vi "Create board.vi"(8 "error in (no error)":errorcluster) -> (0 "error out":errorcluster, 3 "Empty board":refnum<class "Board.lvclass">)   [LabVIEW 2016, in "Chesslib.lvlib" / "Board.lvclass"]
uses:
  Board.lvclass
  Pieces/Piece/Piece.lvclass
  private/Square content.ctl
  Board.lvclass/Board.ctl
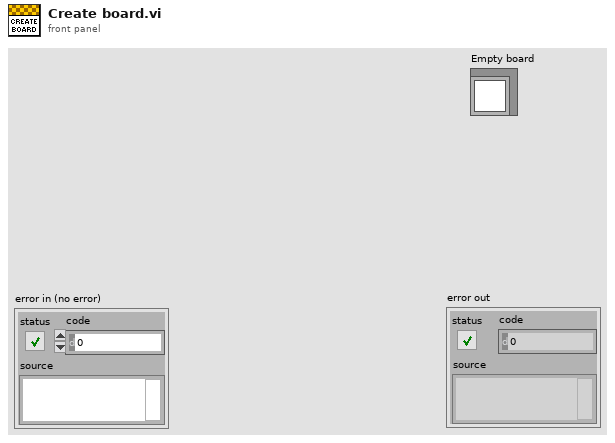
[diagram p1: front panel]
types:
  T1 = typedef "Chesslib.lvlib/Board.lvclass/Square content.ctl" = cluster{"Occupied":bool, "Piece":refnum<class "Piece.lvclass">}
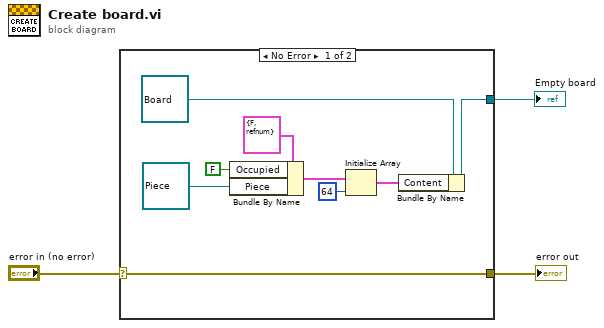
[diagram p0: block diagram]
diagram:
  n1 = case shown="No Error" "error in (no error)" {
    selector: "error in (no error)" -> [w4 w13]
    tunnel: [w6 _] -> w3
    tunnel: [w4 w13] -> w2
    frame No Error {
      n2 = Bundle By Name(cluster=T1 {"Occupied"=FALSE, "Piece"=refnum} ("Square content"), "Occupied"=FALSE, "Piece"=refnum<class "Piece.lvclass"> refnum) -> (w7:T1)
      n3 = Initialize Array(w7, 64 ("dimension size")) -> (w11:T1[])
      n4 = Bundle By Name(cluster=refnum<class "Board.lvclass"> refnum ("Board in"), "Content"=w11) -> (w6:refnum<class "Board.lvclass">)
    }
    frame Error {
    }
  }
  "Empty board" <- w3
  "error out" <- w2
